vi "CCT_Snippet.vi"(8 "error in (no error)":errorcluster, 11 "CCT Instance":T1) -> (0 "error out":errorcluster)   [LabVIEW 2009]
uses:
  DataStructures/CCT_ObjectReference.ctl
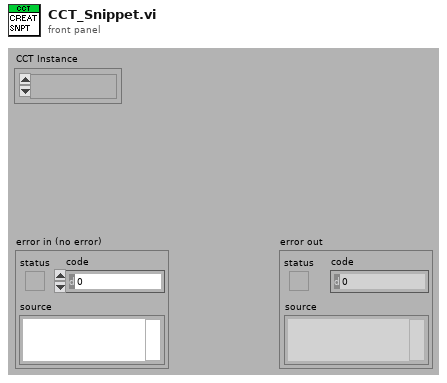
[diagram p1: front panel]
types:
  T1 = typedef "CCT_ObjectReference.ctl" = refnum<k1>
  T2 = cluster{"Year":u16, "Month":u8, "Day":u8, "Hour":u8, "Minute":u8, "Second":u8}
  T3 = enum16{"open", "open or create", "create or replace", "create", "open (read only)"}
  T4 = typedef "CCT_BD Capture Options.ctl" = enum16{"No", "Selected", "Visible", "All"}
  T5 = typedef "CCT_SnippetOptions.ctl" = cluster{"CreateSnippet":bool, "SnippetHeader":string, "EmbeddedHeader":string, "HeaderColor":u32, "Version":string}
  T6 = enum16{"open", "replace", "create", "open or create", "replace or create", "replace or create with confirmation"}
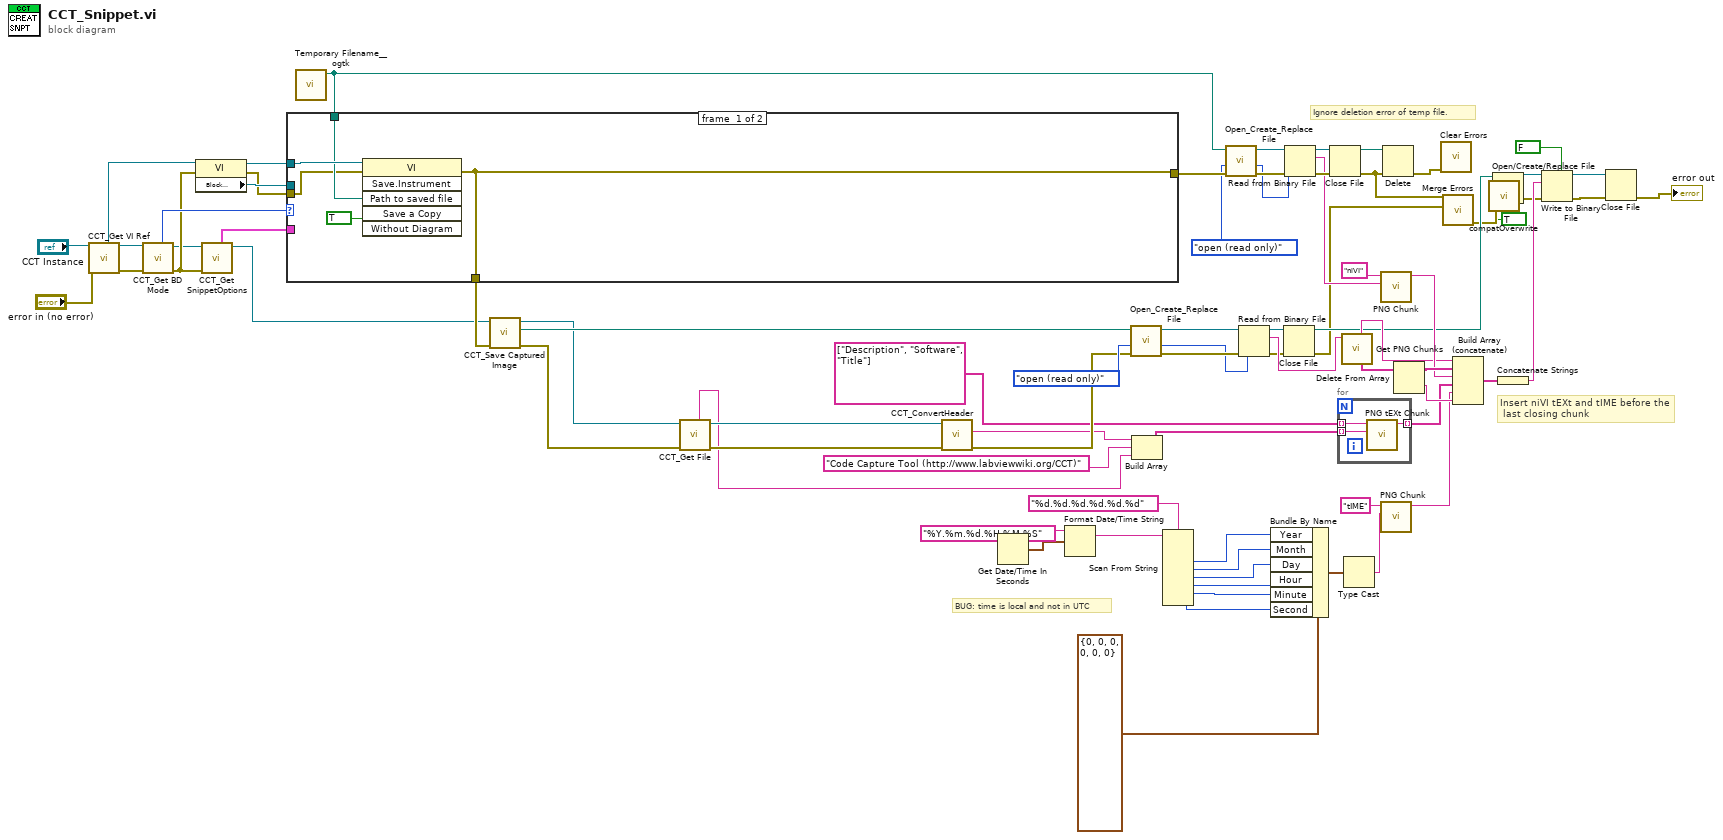
[diagram p0: block diagram]
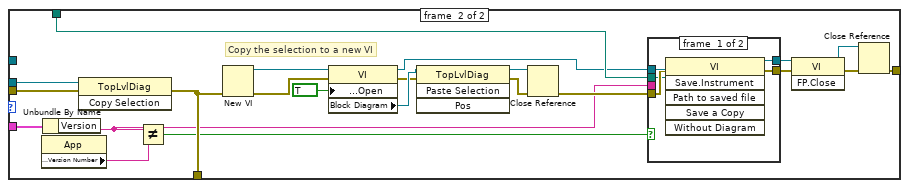
[diagram p2: hidden frame]
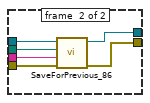
[diagram p3: hidden frame]
diagram:
  # "Ignore deletion error of temp file."
  # "Insert niVI tEXt and tIME before the\n last closing chunk"
  # "BUG: time is local and not in UTC"
  n1 = call "CCT_Get VI Ref.vi"("error in (no error)"="error in (no error)", "reference"="CCT Instance") -> ("error out"=w22:errorcluster, "duplicate reference"=w23:T1, "VI To Capture"=w24:refnum<vi>)  [unwired: 7 in]
  n2 = call "CCT_Get BD Mode.vi"("error in (no error)"=w22, "reference"=w23) -> ("error out"=w6:errorcluster, "duplicate reference"=w5:T1, "BD Mode"=w16:T4)  [unwired: 7 in]
  n3 = property class="VI"(reference=w24, error in=w6) -> (reference out=w15:refnum<vi>, error out=w20:errorcluster, "Block Diagram"=w21:refnum<vi>)
  n4 = call "CCT_Get SnippetOptions.vi"("error in (no error)"=w6, "reference"=w5) -> ("duplicate reference"=w4:T1, "SnippetOptions"=w3:T5)  [unwired: 7 in, 1 out]
  n5 = call <userlib>:"Temporary Filename__ogtk.vi"() -> ("file in tmp dir"=w14:path)  [unwired: 6 in, 1 out]
  n6 = case shown="Default" w16 {
    tunnel: [w81 w96] -> w77
    tunnel: w21 -> [_ w95]
    tunnel: w20 -> [w80 w94]
    tunnel: [w81 w93] -> w19
    tunnel: w15 -> [w84 _]
    tunnel: w14 -> [w82 w90]
    tunnel: w3 -> [_ w89]
    frame #0 {
      n7 = invoke class="VI" method="Save.Instrument"(reference=w84, error in=w80, "Path to saved file"=w82, "Save a Copy"=TRUE) -> (error out=w81:errorcluster)  [unwired: 2 in, 5 out]
    }
    frame #1 {
      # "Copy the selection to a new VI"
      n8 = property class="App"() -> ("Application:Version Number"=w88:string)  [unwired: 2 in, 2 out]
      n9 = Unbundle By Name(w89) -> ("Version"=w86:string)
      n10 = invoke class="TopLvlDiag" method="Copy Selection"(reference=w95, error in=w94) -> (error out=w93:errorcluster)  [unwired: 1 in, 2 out]
      n11 = Not Equal?(x=w86, y=w88) -> (x != y?=w87:bool)
      n12 = New VI(8:w93) -> (0:w102:errorcluster, 3:w92:refnum<vi>)  [unwired: 6 in]
      n13 = property class="VI"(reference=w92, error in=w102, "Block Diagram Window:Open"=TRUE) -> (reference out=w85:refnum<vi>, error out=w104:errorcluster, "Block Diagram"=w105:refnum<vi>)
      n14 = invoke class="TopLvlDiag" method="Paste Selection"(reference=w105, error in=w104) -> (reference out=w103:refnum<vi>, error out=w101:errorcluster)  [unwired: 2 in, 2 out]
      n15 = Close Reference(reference=w103, error in (no error)=w101) -> (error out=w91:errorcluster)
      n16 = case shown="True" w87 {
        tunnel: w85 -> [w111 w113]
        tunnel: [w110 w112] -> w100
        tunnel: [w109 w117] -> w99
        tunnel: w91 -> [w108 w116]
        tunnel: w90 -> [w107 w114]
        tunnel: w86 -> [_ w115]
        frame #0 {
          n17 = invoke class="VI" method="Save.Instrument"(reference=w111, error in=w108, "Path to saved file"=w107) -> (reference out=w110:refnum<vi>, error out=w109:errorcluster)  [unwired: 3 in, 4 out]
        }
        frame #1 {
          n18 = call "SaveForPrevious_86.vi"("error in (no error)"=w116, "Target Version"=w115, "VI Path"=w114, "VI Refnum In"=w113) -> ("error out"=w117:errorcluster, "VI Refnum Out"=w112:refnum<vi>)  [unwired: 6 in]
        }
      }
      n19 = invoke class="VI" method="FP.Close"(reference=w100, error in=w99) -> (reference out=w97:refnum<vi>, error out=w98:errorcluster)  [unwired: 1 in, 1 out]
      n20 = Close Reference(reference=w97, error in (no error)=w98) -> (error out=w96:errorcluster)
    }
  }
  n21 = call "CCT_Save Captured Image.vi"("error in (no error)"=w19, "reference"=w4) -> ("error out"=w18:errorcluster, "Created File"=w52:path, "duplicate reference"=w12:T1)  [unwired: 7 in]
  n22 = call "CCT_Get File.vi"("error in (no error)"=w18, "reference"=w12) -> ("error out"=w17:errorcluster, "duplicate reference"=w11:T1, "File Name"=w10:string)  [unwired: 7 in]
  n23 = call "CCT_ConvertHeader.vi"("error out"=w17, "reference"=w11) -> ("error in (no error)"=w49:errorcluster, "Embedded Info"=w33:string)  [unwired: 7 in, 1 out]
  n24 = Get Date/Time In Seconds() -> (seconds since 1Jan1904=w44:timestamp)
  n25 = Format Date/Time String(time format string (%c)="%Y.%m.%d.%H.%M.%S", seconds (now)=w44) -> (date/time string=w42:string)  [unwired: 1 in]
  n26 = call <vilib>:"Open_Create_Replace File.vi"("error in (no error)"=w49, "function (open:0)"=T3."open (read only)", "file path"=w52) -> ("error out"=w60:errorcluster, "file size (bytes)"=w25:i32, "refnum"=w59:refnum<file>)  [unwired: 5 in, 1 out]
  n27 = Build Array(w33, "Code Capture Tool (http://www.labviewwiki.org/CCT)", w10) -> (w31:string[])
  n28 = Scan From String(format string="%d.%d.%d.%d.%d.%d", input string=w42) -> (output 1=w40:i32, output 2=w39:i32, output 3=w38:i32, output 4=w37:i32, output 5=w36:i32, output 6=w35:i32)  [unwired: 8 in, 3 out]
  n29 = call <vilib>:"Open_Create_Replace File.vi"("error in (no error)"=w77, "function (open:0)"=T3."open (read only)", "file path"=w14) -> ("error out"=w57:errorcluster, "file size (bytes)"=w55:i32, "refnum"=w56:refnum<file>)  [unwired: 5 in, 1 out]
  n30 = Read from Binary File(8:w60, 10:w25, 11:w59) -> (0:w62:errorcluster, 2:w66:string, 3:w63:refnum<file>)  [unwired: 3 in, 1 out]
  n31 = Bundle By Name(cluster=T2 {"Year"=0, "Month"=0, "Day"=0, "Hour"=0, "Minute"=0, "Second"=0}, "Year"=w40, "Month"=w39, "Day"=w38, "Hour"=w37, "Minute"=w36, "Second"=w35) -> (w45:T2)
  n32 = Close File(refnum=w63, error in=w62) -> (path=w29:path, error out=w7:errorcluster)
  n33 = Read from Binary File(8:w57, 10:w55, 11:w56) -> (0:w78:errorcluster, 2:w74:string, 3:w79:refnum<file>)  [unwired: 3 in, 1 out]
  n34 = Close File(refnum=w79, error in=w78) -> (path=w76:path, error out=w9:errorcluster)
  n35 = for {
    tunnel: [w120] -> w53 mode=indexing
    tunnel: w31 -> [w119] mode=indexing
    tunnel: string[] ["Description", "Software", "Title"] -> [w118] mode=indexing
    n36 = call "PNG tEXt Chunk.vi"("Contents"=w119, "Keyword"=w118) -> ("PNG Chunk"=w120:string)  [unwired: 9 in]
  }
  n37 = call "Get PNG Chunks.vi"("data"=w66) -> ("Chunks"=w73:string[], "Header"=w65:string)  [unwired: 5 in, 4 out]
  n38 = Type Cast(x=w45) -> (*(type *) &x=w46:string)  [unwired: 1 in]
  n39 = call "PNG Chunk.vi"("Data"=w74, "Name"="niVI" ("element")) -> ("PNG Chunk"=w71:string)  [unwired: 9 in]
  n40 = call "PNG Chunk.vi"("Data"=w46, "Name"="tIME") -> ("PNG Chunk"=w48:string)  [unwired: 9 in]
  n41 = Delete(path (use dialog)=w76, error in=w9) -> (error out=w8:errorcluster)  [unwired: 3 in, 2 out]
  n42 = Delete From Array(array=w73) -> (deleted portion=w54:string, array with subset deleted=w72:string[])  [unwired: 2 in]
  n43 = call <vilib>:"Clear Errors.vi"("error in (no error)"=w8) -> ()  [unwired: 6 in, 1 out]
  n44 = call <vilib>:"Merge Errors.vi"("error in 2 (no error)"=w7, "error in 1 (no error)"=w9) -> ("error out"=w28:errorcluster)  [unwired: 5 in]
  n45 = Build Array (concatenate)(w65, w72, w71, w53, w48, w54) -> (w68:string[])
  n46 = call <vilib>:"compatOverwrite.vi"("overwrite (F)"=TRUE ("advisory dialog? (display:T)")) -> ("overwrite?"=w2:T6)
  n47 = Open/Create/Replace File(file path (use dialog)=w29, error in=w28, operation (0:open)=w2) -> (refnum out=w30:refnum<file>, error out=w27:errorcluster)  [unwired: 3 in, 1 out]
  n48 = Concatenate Strings(w68) -> (w64:string)
  n49 = Write to Binary File ("Write File")(file (use dialog)=w30, data=w64, error in=w27, 5:FALSE ("prepend array or string size? (T)")) -> (refnum out=w69:refnum<file>, error out=w70:errorcluster)  [unwired: 2 in, 1 out]
  n50 = Close File(refnum=w69, error in=w70) -> (error out=→"error out":errorcluster)  [unwired: 1 out]
